vi "Actor Core.vi"(8 "error in":errorcluster, 11 "Test Channel View in":refnum<class "HVAC System View.lvclass">) -> (0 "error out":errorcluster, 3 "Actor out":refnum<class "Actor.lvclass">)   [LabVIEW 2013, in "HVAC System View.lvlib" / "HVAC System View.lvclass"]
doc: "(<B>Filename</B>: Actor Framework.lvlib:Actor.lvclass:Actor Core.vi)\n\nReceives messages to the actor, reacts to them, and initiates any error handling that may shut the actor down.\n\nDescendant classes may override this VI to append parallel tasks for the actor to complete while it handles messages. Overrides use the Call Parent Method node."
uses:
  HVAC System View.lvclass
  <vilib>/ActorFramework/Actor/Actor.lvclass
  Resources/UI Controls/Test Item Tiles.ctl
  Resources/UI Controls/Test Item Tile.ctl
  Resources/UI Controls/Delete Frame.ctl
  HVAC System View.lvclass/HVAC System View.ctl
  <vilib>/ActorFramework/Actor/Actor.lvclass/Actor.ctl
  <vilib>/ActorFrameworkMVC/View Actor/View Actor.lvclass
  <vilib>/ActorFramework/Message Enqueuer/Message Enqueuer.lvclass/Message Enqueuer.ctl
  HVAC System View Messages/Update Tiles Msg/Update Tiles Msg.lvclass/Update Tiles Msg.ctl
  <vilib>/Utility/miscctls.llb/LVPositionTypeDef.ctl
  <vilib>/ActorFrameworkMVC/UI Controller Messages/Move Subpanel Msg/Move Subpanel Msg.lvclass/Move Subpanel Msg.ctl
  <vilib>/ActorFrameworkMVC/UI Controller Messages/Insert Subpanel Msg/Insert Subpanel Msg.lvclass/Insert Subpanel Msg.ctl
  <vilib>/ActorFrameworkMVC/UI Controller Messages/Move Splitter Msg/Move Splitter Msg.lvclass/Move Splitter Msg.ctl
  <vilib>/ActorFramework/Message Enqueuer/Init from Existing Queue.vi
  <vilib>/ActorFramework/Message Enqueuer/Enqueue.vi
  <vilib>/ActorFramework/Message Priority Queue/Priority Enqueue.vi
  <vilib>/ActorFramework/Message Enqueuer/Message Enqueuer.lvclass
  HVAC System View Messages/Update Tiles Msg/Update Tiles Msg.lvclass
  HVAC System View Messages/Move In Previous Page Msg/Move In Previous Page Msg.lvclass
  HVAC System View Messages/Move In Next Page Msg/Move In Next Page Msg.lvclass
  <vilib>/ActorFrameworkMVC/UI Controller Messages/Move Subpanel Msg/Move Subpanel Msg.lvclass
  <vilib>/ActorFrameworkMVC/UI Controller Messages/Insert Subpanel Msg/Insert Subpanel Msg.lvclass
  Models/Project Model Messages/Preview Project Msg/Preview Project Msg.lvclass
  Models/Project Model Messages/Update Tiles Info Msg/Update Tiles Info Msg.lvclass
  Models/Project Model Messages/Update Previous Button Visibility Msg/Update Previous Button Visibility Msg.lvclass
  Models/Project Model Messages/Update Next Button Visibility Msg/Update Next Button Visibility Msg.lvclass
  HVAC System View Messages/Move Out Next Page Msg/Move Out Next Page Msg.lvclass
  Models/HVAC System Model Messages/Next Page Msg/Next Page Msg.lvclass
  HVAC System View Messages/Move Out Previous Page Msg/Move Out Previous Page Msg.lvclass
  Models/HVAC System Model Messages/Previous Page Msg/Previous Page Msg.lvclass
  <vilib>/ActorFrameworkMVC/UI Controller Messages/Move Splitter Msg/Move Splitter Msg.lvclass
  <vilib>/ActorFrameworkMVC/View Actor Messages/Get Model Enqueuer Msg/Get Model Enqueuer Msg.lvclass
  <vilib>/ActorFrameworkMVC/UI Controller Messages/Get Model Actor Enqueuer Msg/Get Model Actor Enqueuer Msg.lvclass
panel:
  in  "Frame":T1
  in  "Previous Button":bool
  in  "Next Button":bool
  out "Tiles":T2
  in  "Back":bool
  # "暖通空调系统性能检测"
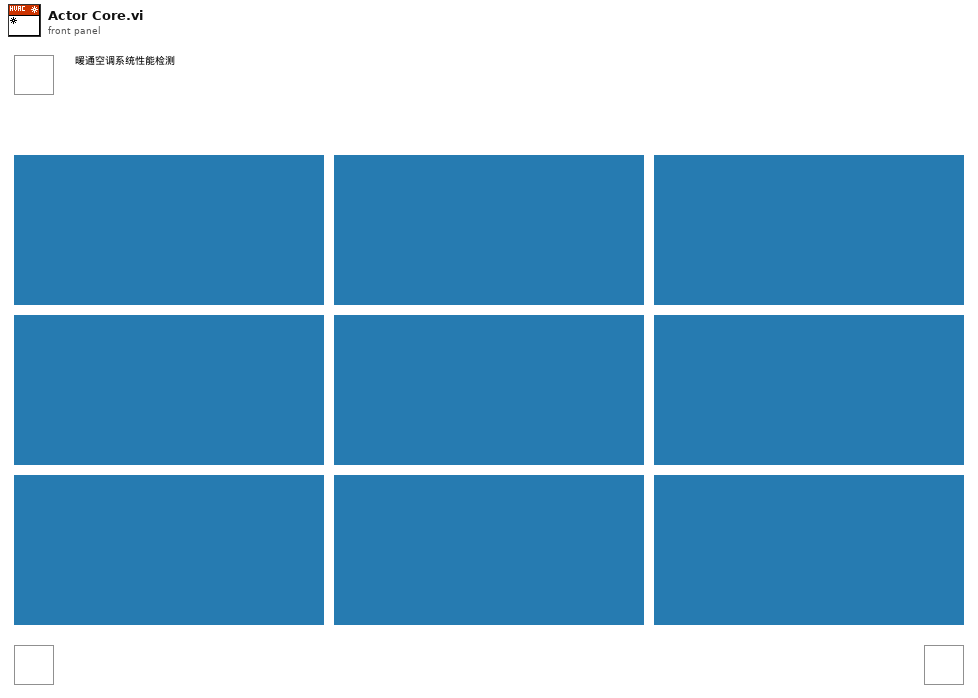
[diagram p1: front panel]
types:
  T1 = typedef "Delete Frame.ctl" = bool
  T2 = typedef "Test Item Tiles.ctl" = cluster{"Tile 1":T3, "Tile 2":T3, "Tile 3":T3, "Tile 4":T3, "Tile 5":T3, "Tile 6":T3, "Tile 7":T3, "Tile 8":T3, "Tile 9":T3}
  T3 = typedef "Test Item Tile.ctl" = cluster{"Name":string, "View":string, "Mode":string}
  T4 = typedef "HVAC System View.lvlib/HVAC System View.lvclass/Events.ctl" = cluster{"Update Tiles Info":refnum<user-event>, "Set Previous Button Visibility":refnum<user-event>, "Set Next Button Visibility":refnum<user-event>, "Move In Previous":refnum<user-event>, "Move In Next":refnum<user-event>}
  T5 = typedef "LVPositionTypeDef.ctl" = cluster{"Left":i32, "Top":i32}
  T6 = enum8{"Enabled", "Disabled", "Disabled and Grayed Out"}
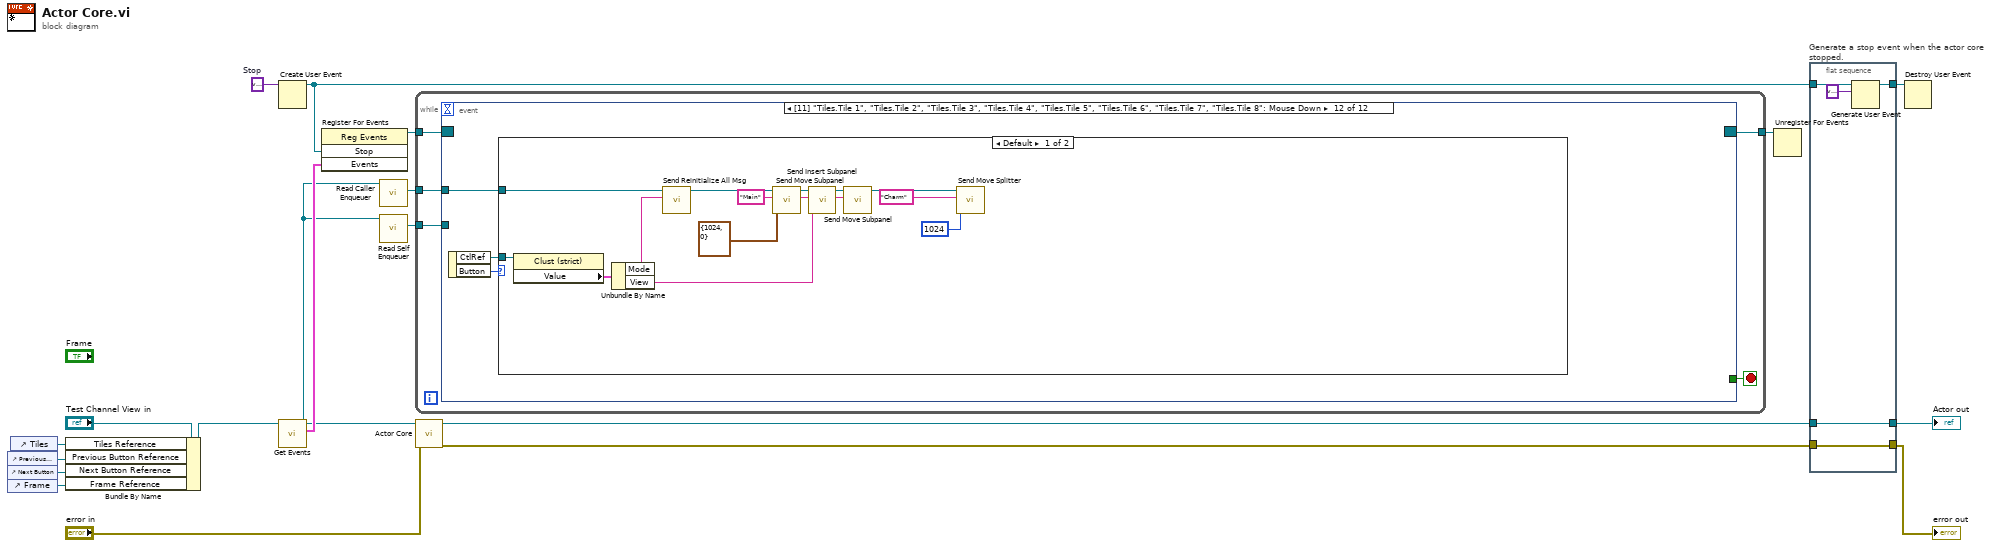
[diagram p0: block diagram]
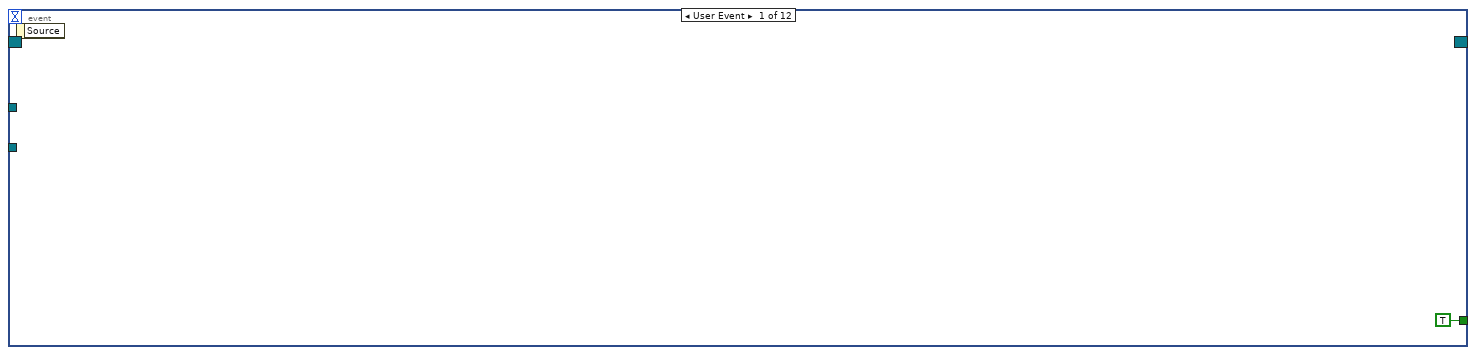
[diagram p2: hidden frame]
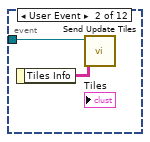
[diagram p3: hidden frame]
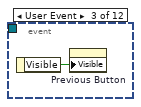
[diagram p4: hidden frame]
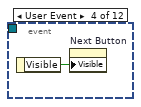
[diagram p5: hidden frame]
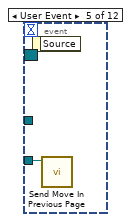
[diagram p6: hidden frame]
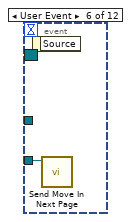
[diagram p7: hidden frame]
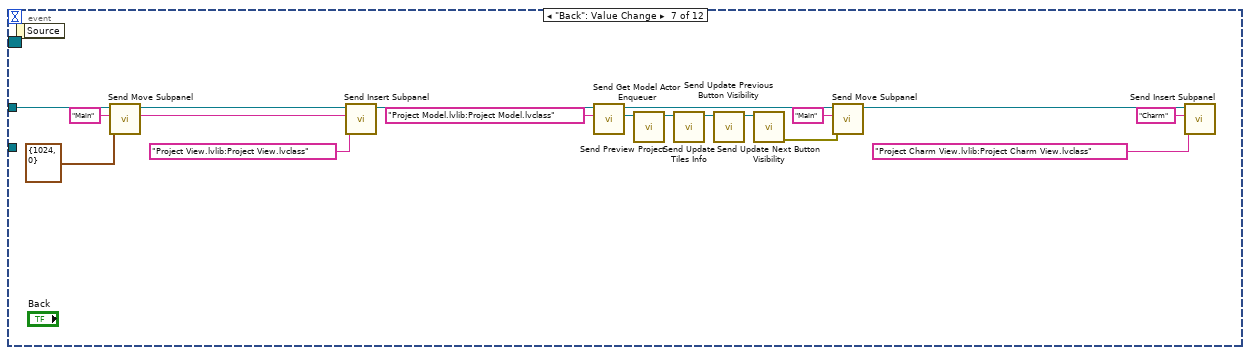
[diagram p8: hidden frame]
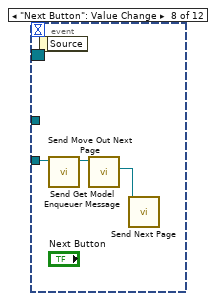
[diagram p9: hidden frame]
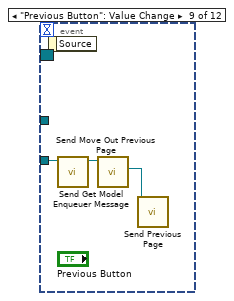
[diagram p10: hidden frame]
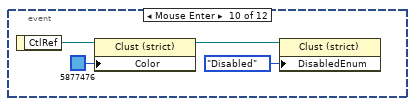
[diagram p11: hidden frame]
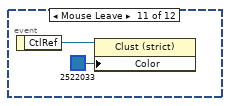
[diagram p12: hidden frame]
diagram:
  w20 = variant  # Stop
  n1 = control-ref of="Previous Button"() -> (w5:refnum<vi>)
  n2 = control-ref of="Next Button"() -> (w6:refnum<vi>)
  n3 = control-ref of="Frame"() -> (w7:refnum<vi>)
  n4 = control-ref of="Tiles"() -> (w1:refnum<vi>)
  n5 = Bundle By Name(cluster="Test Channel View in", "Tiles Reference"=w1, "Previous Button Reference"=w5, "Next Button Reference"=w6, "Frame Reference"=w7) -> (w8:refnum<class "HVAC System View.lvclass">)
  n6 = Create User Event(user event datatype=w20) -> (user event=w11:refnum<user-event>)  [unwired: 1 in, 1 out]
  n7 = call "Get Events.vi"("Test Channel View in"=w8) -> ("Events"=w10:T4, "Test Channel View out"=w4:refnum<class "HVAC System View.lvclass">)  [unwired: 9 in]
  n8 = register-events(w11, w10) -> (reference out=w12:refnum<event-registration>)  [unwired: 2 in, 1 out]
  n9 = call <vilib>:"Read Caller Enqueuer.vi"("Actor"=w4) -> ("Caller Enqueuer"=w3:refnum<class "Message Enqueuer.lvclass">)  [unwired: 10 in]
  n10 = call <vilib>:"Read Self Enqueuer.vi"("Actor"=w4) -> ("Self Enqueuer"=w2:refnum<class "Message Enqueuer.lvclass">)  [unwired: 10 in]
  n11 = while {
    tunnel: [w25] -> w9
    tunnel: w12 -> [w23]
    tunnel: w3 -> [w22]
    tunnel: w2 -> [w21]
    stop <- w24 stop-if-true
    n12 = event shown="[11] \"Tiles.Tile 1\", \"Tiles.Tile 2\", \"Tiles.Tile 3\", \"Tiles.Tile 4\", \"Tiles.Tile 5\", \"Tiles.Tile 6\", \"Tiles.Tile 7\", \"Tiles.Tile 8\": Mouse Down" {
      selector: w23 -> [_ _ _ _ _ _ _ _ _ _ _ _]
      dyn-events: [_ _ _ _ _ _ _ _ _ _ _ _] -> w25
      timeout: _ -> [_ _ _ _ _ _ _ _ _ _ _ _]
      tunnel: [TRUE _ _ _ _ _ _ _ _ _ _ _] -> w24
      tunnel: w22 -> [_ _ _ _ _ _ w33 _ _ _ _ w62]
      tunnel: w21 -> [_ w27 _ _ w31 w32 _ w51 w54 _ _ _]
      event User Event {
        n13 = event-data() -> ()  [unwired: 1 in, 1 out]
      }
      event User Event {
        n14 = event-data() -> ("Tiles Info"=w28:string[][])  [unwired: 1 in]
        n15 = call "Send Update Tiles.vi"("Channel Tiles Info"=w28, "Message Enqueuer"=w27) -> ()  [unwired: 8 in, 2 out]
      }
      event User Event {
        n16 = event-data() -> ("Visible"=w29:bool)  [unwired: 1 in]
        n17 = property on="Previous Button" class="Bool"("Visible"=w29) -> ()  [unwired: 2 in, 2 out]
      }
      event User Event {
        n18 = event-data() -> ("Visible"=w30:bool)  [unwired: 1 in]
        n19 = property on="Next Button" class="Bool"("Visible"=w30) -> ()  [unwired: 2 in, 2 out]
      }
      event User Event {
        n20 = event-data() -> ()  [unwired: 1 in, 1 out]
        n21 = call "Send Move In Previous Page.vi"("Message Enqueuer"=w31) -> ()  [unwired: 9 in, 2 out]
      }
      event User Event {
        n22 = event-data() -> ()  [unwired: 1 in, 1 out]
        n23 = call "Send Move In Next Page.vi"("Message Enqueuer"=w32) -> ()  [unwired: 9 in, 2 out]
      }
      event "Back": Value Change {
        w46 = "Main" ("Subpanel Name")
        n24 = event-data() -> ()  [unwired: 1 in, 1 out]
        n25 = call <vilib>:"Send Move Subpanel.vi"("Position (0,0)"=T5 {"Left"=1024, "Top"=0}, "Subpanel Name"=w46, "Message Enqueuer"=w33) -> ("Message Enqueuer out"=w49:refnum<class "Message Enqueuer.lvclass">)  [unwired: 7 in, 1 out]
        n26 = call <vilib>:"Send Insert Subpanel.vi"("View Name"="Project View.lvlib:Project View.lvclass" ("Subpanel Name"), "Subpanel Name"=w46, "Message Enqueuer"=w49) -> ("Message Enqueuer out"=w43:refnum<class "Message Enqueuer.lvclass">)  [unwired: 7 in, 1 out]
        n27 = call <vilib>:"Send Get Model Actor Enqueuer.vi"("Model Name"="Project Model.lvlib:Project Model.lvclass", "Message Enqueuer in"=w43) -> ("Reply"=w34:refnum<class "Message Enqueuer.lvclass">, "Message Enqueuer out"=w42:refnum<class "Message Enqueuer.lvclass">)  [unwired: 6 in, 2 out]
        n28 = call "Send Preview Project.vi"("Message Enqueuer"=w34) -> ("Message Enqueuer out"=w44:refnum<class "Message Enqueuer.lvclass">)  [unwired: 9 in, 1 out]
        n29 = call "Send Update Tiles Info.vi"("Message Enqueuer"=w44) -> ("Message Enqueuer out"=w40:refnum<class "Message Enqueuer.lvclass">)  [unwired: 9 in, 1 out]
        n30 = call "Send Update Previous Button Visibility.vi"("Message Enqueuer"=w40) -> ("Message Enqueuer out"=w39:refnum<class "Message Enqueuer.lvclass">)  [unwired: 9 in, 1 out]
        n31 = call "Send Update Next Button Visibility.vi"("Message Enqueuer"=w39) -> ("error out"=w38:errorcluster)  [unwired: 9 in, 1 out]
        n32 = call <vilib>:"Send Move Subpanel.vi"("error in (no error)"=w38, "Subpanel Name"="Main", "Message Enqueuer"=w42) -> ("Message Enqueuer out"=w37:refnum<class "Message Enqueuer.lvclass">)  [unwired: 7 in, 1 out]
        n33 = call <vilib>:"Send Insert Subpanel.vi"("View Name"="Project Charm View.lvlib:Project Charm View.lvclass", "Subpanel Name"="Charm", "Message Enqueuer"=w37) -> ()  [unwired: 7 in, 2 out]
      }
      event "Next Button": Value Change {
        n34 = event-data() -> ()  [unwired: 1 in, 1 out]
        n35 = call "Send Move Out Next Page.vi"("Message Enqueuer"=w51) -> ("Message Enqueuer out"=w50:refnum<class "Message Enqueuer.lvclass">)  [unwired: 9 in, 1 out]
        n36 = call <vilib>:"Send Get Model Enqueuer Message.vi"("Message Enqueuer in"=w50) -> ("Reply"=w52:refnum<class "Message Enqueuer.lvclass">)  [unwired: 7 in, 3 out]
        n37 = call "Send Next Page.vi"("Message Enqueuer"=w52) -> ()  [unwired: 9 in, 2 out]
      }
      event "Previous Button": Value Change {
        n38 = event-data() -> ()  [unwired: 1 in, 1 out]
        n39 = call "Send Move Out Previous Page.vi"("Message Enqueuer"=w54) -> ("Message Enqueuer out"=w53:refnum<class "Message Enqueuer.lvclass">)  [unwired: 9 in, 1 out]
        n40 = call <vilib>:"Send Get Model Enqueuer Message.vi"("Message Enqueuer in"=w53) -> ("Reply"=w55:refnum<class "Message Enqueuer.lvclass">)  [unwired: 7 in, 3 out]
        n41 = call "Send Previous Page.vi"("Message Enqueuer"=w55) -> ()  [unwired: 9 in, 2 out]
      }
      event Mouse Enter {
        n42 = event-data() -> ("CtlRef"=w56:refnum<vi>)  [unwired: 1 in]
        n43 = property class="Clust (strict)"(reference=w56, "Color"=u32 5877476) -> (reference out=w58:refnum<vi>)  [unwired: 1 in, 1 out]
        n44 = property class="Clust (strict)"(reference=w58, "DisabledEnum"=T6."Disabled" ("Disabled")) -> ()  [unwired: 1 in, 2 out]
      }
      event Mouse Leave {
        n45 = event-data() -> ("CtlRef"=w60:refnum<vi>)  [unwired: 1 in]
        n46 = property class="Clust (strict)"(reference=w60, "Color"=u32 2522033) -> ()  [unwired: 1 in, 2 out]
      }
      event Mouse Down {
        n47 = event-data() -> ("CtlRef"=w64:refnum<vi>, "Button"=w63:u16)  [unwired: 1 in]
        n48 = case shown="Default" w63 {
          tunnel: w64 -> [w76 _]
          tunnel: w62 -> [w77 _]
          frame Default {
            w72 = "Main" ("Subpanel Name")
            n49 = property class="Clust (strict)"(reference=w76) -> ("Value"=w67:T3)  [unwired: 1 in, 2 out]
            n50 = Unbundle By Name(w67) -> ("Mode"=w65:string, "View"=w66:string)
            n51 = call "Send Reinitialize All Msg.vi"("Mode"=w65, "Message Enqueuer in"=w77) -> ("Message Enqueuer out"=w68:refnum<class "Message Enqueuer.lvclass">)  [unwired: 9 in]
            n52 = call <vilib>:"Send Move Subpanel.vi"("Position (0,0)"=T5 {"Left"=1024, "Top"=0}, "Subpanel Name"=w72, "Message Enqueuer"=w68) -> ("Message Enqueuer out"=w69:refnum<class "Message Enqueuer.lvclass">)  [unwired: 7 in, 1 out]
            n53 = call <vilib>:"Send Insert Subpanel.vi"("View Name"=w66, "Subpanel Name"=w72, "Message Enqueuer"=w69) -> ("Message Enqueuer out"=w71:refnum<class "Message Enqueuer.lvclass">)  [unwired: 7 in, 1 out]
            n54 = call <vilib>:"Send Move Subpanel.vi"("Subpanel Name"=w72, "Message Enqueuer"=w71) -> ("Message Enqueuer out"=w73:refnum<class "Message Enqueuer.lvclass">)  [unwired: 8 in, 1 out]
            n55 = call <vilib>:"Send Move Splitter.vi"("Splitter Position"=1024, "Splitter Name"="Charm", "Message Enqueuer"=w73) -> ()  [unwired: 7 in, 2 out]
          }
          frame 2 {
          }
        }
      }
    }
  }
  n56 = call-parent "Actor Core.vi"("error in"="error in", "View Actor in"=w4) -> ("error out"=w15:errorcluster, "Actor out"=w16:refnum<class "Actor.lvclass">)  [unwired: 8 in]
  n57 = Unregister For Events(event registration refnum=w9) -> ()  [unwired: 1 in, 1 out]
  n58 = flat-sequence "Generate a stop event when the actor core stopped." {
    tunnel: w11 -> [w82]
    tunnel: [w80] -> w19
    tunnel: w16 -> [w79]
    tunnel: w15 -> [w78]
    tunnel: [w79] -> w14
    tunnel: [w78] -> w13
    frame #0 {
      n59 = Generate User Event(user event=w82, event data cluster=variant ("event data")) -> (user event out=w80:refnum<user-event>)  [unwired: 2 in, 1 out]
    }
  }
  n60 = Destroy User Event(user event=w19) -> ()  [unwired: 1 in, 1 out]
  "error out" <- w13
  "Actor out" <- w14
